vi "TRIG_conf2.vi"() -> ()   [LabVIEW 2012]
uses:
  global.vi
  <vilib>/Platform/browser.llb/Open URL in Default Browser (string).vi
panel:
  in  "additional_time":dbl=5e-06
  out "trig inhibit":dbl=100.0 min=0.0 max=999.999999999995 format="%.2p"
  out "exp cycle":dbl=100.0 min=0.0 max=999.999999999995 format="%.2f"
  out "delay cycle":dbl=100.0 min=0.0 max=999.999999999995 format="%.2f"
  in  "Close":bool
  in  "Reset TRIG":bool
  in  "write config":bool
  in  "BG cycle":dbl=100.0 format="%.2f"
  in  "mol. delay":dbl=100.0 min=0.0 max=999.999999999995 format="%.2f"
  out "Burst enable":bool=TRUE caption="Burst"
  out "Digital Waveform Graph":digitalwaveform(graph)={"t0"=timestamp(0 s since 1904-01-01), "dt"=3e-08, "Y"={"transitions"=[], "data"=array4950x4[19800 elements]}}
  in  "burst period":dbl=49.99999999999998 min=1e-07 format="%.2f"
  in  "bursts":i32=3 min=1
  in  "duration":dbl[](array[numeric])=[5.65, 5.0, 40.0, 5.0] min=0.0 format="%.3f"
  in  "start time":dbl[](array[numeric])=[0.0, 1.1, 6.6000000000000005, 6.3999999999999995] format="%.3f"
  in  "time unit":enum16{"s", "ms", "us", "ns"}(ring)=enum."us"
  in  "help":bool
  out "update front panel":bool
  # "Configure Delay Generator (TRIG)"
  # "power AMP"
  # "AWG"
  # "SWITCH"
  # "OSC"
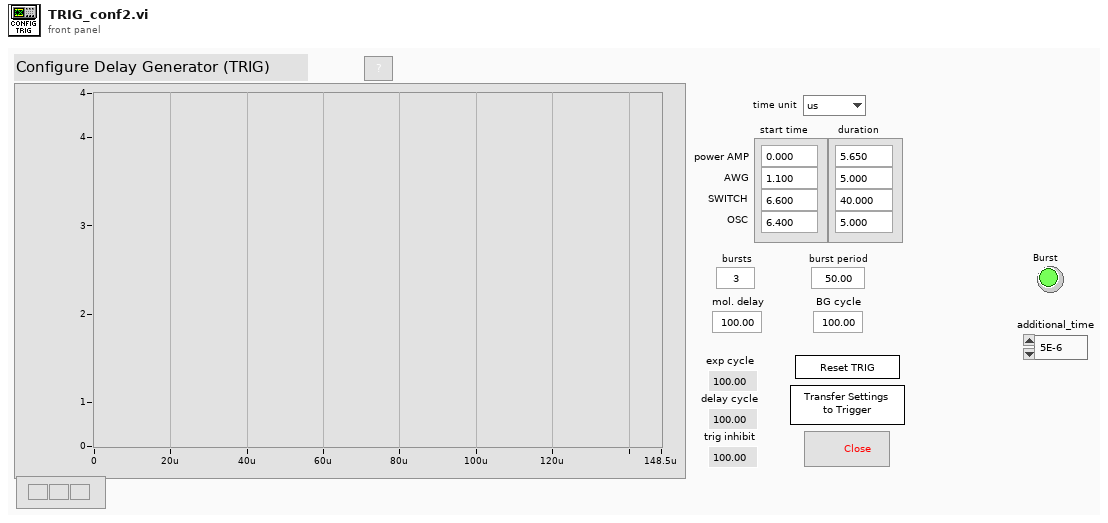
[diagram p1: front panel]
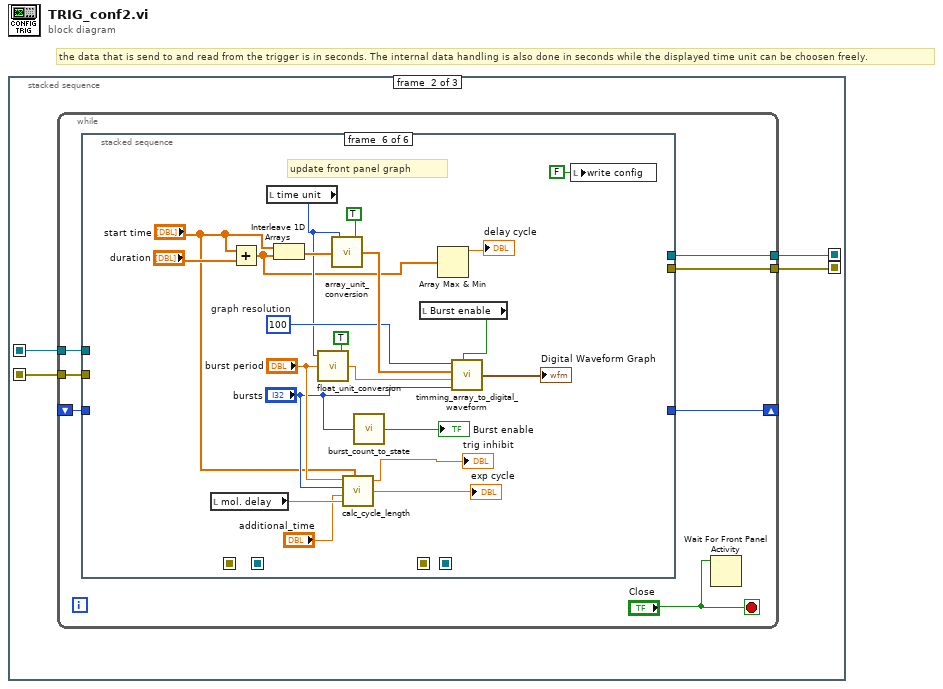
[diagram p0: block diagram]
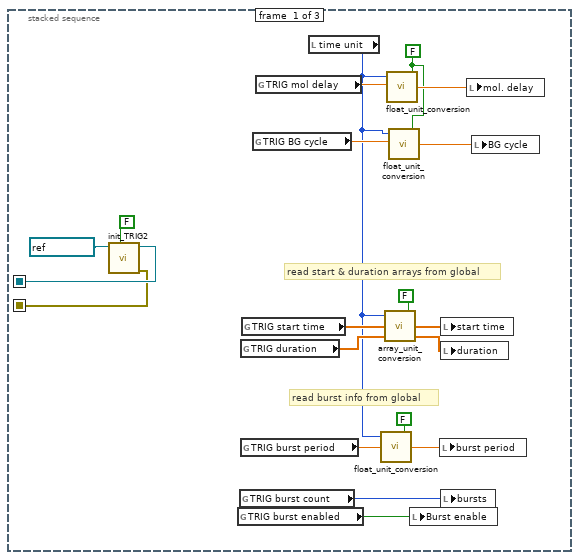
[diagram p2: hidden frame]
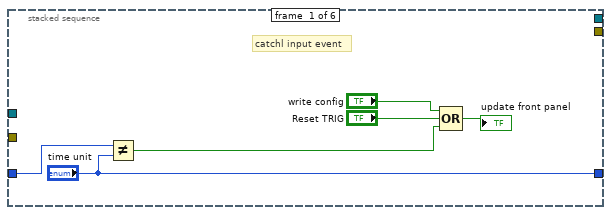
[diagram p3: hidden frame]
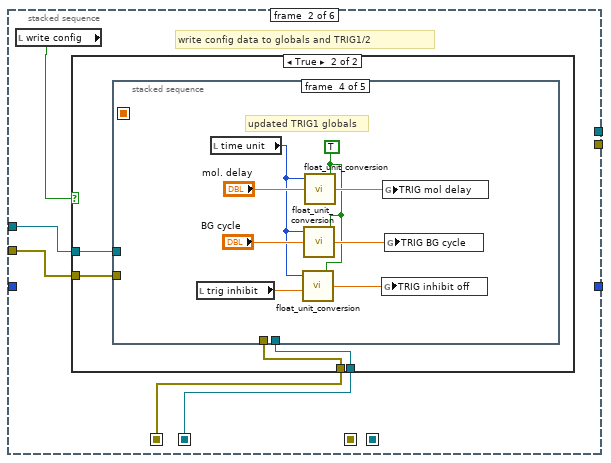
[diagram p4: hidden frame]
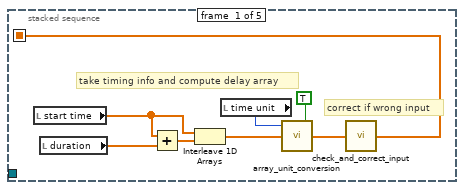
[diagram p6: hidden frame]
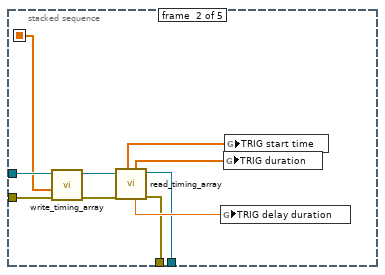
[diagram p7: hidden frame]
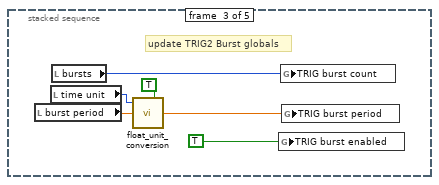
[diagram p8: hidden frame]
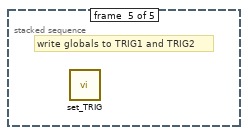
[diagram p9: hidden frame]
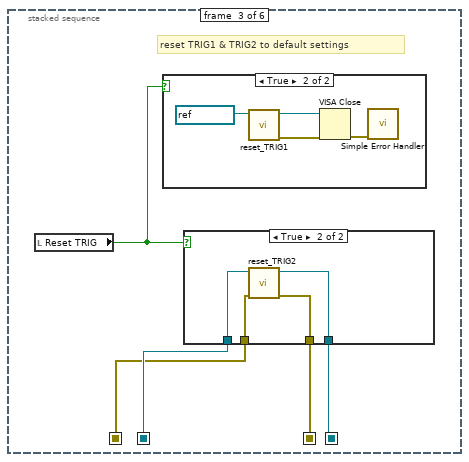
[diagram p10: hidden frame]
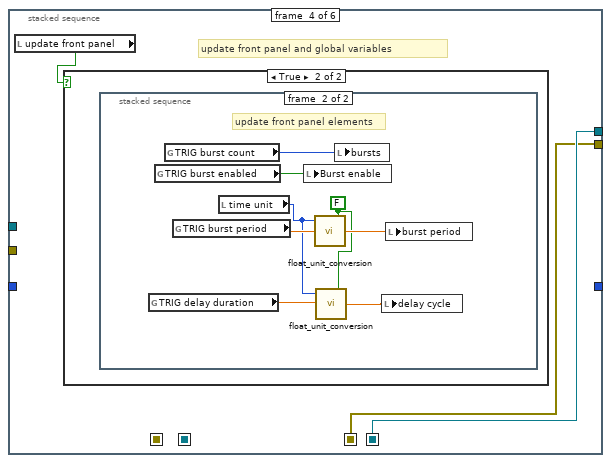
[diagram p13: hidden frame]
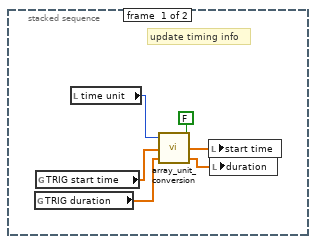
[diagram p15: hidden frame]
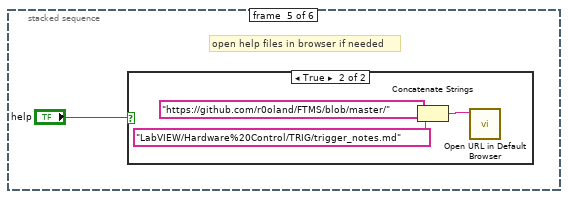
[diagram p16: hidden frame]
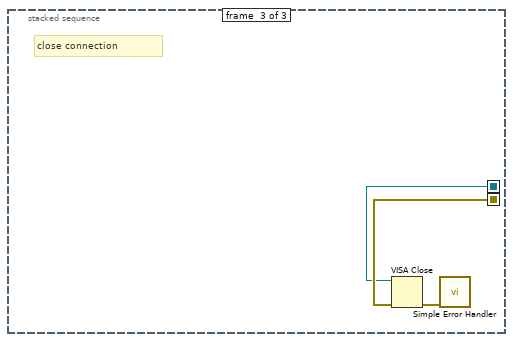
[diagram p18: hidden frame]
diagram:
  # "the data that is send to and read from the trigger is in seconds. The internal data handling is also done in seconds while the displayed time unit can be choosen freely."
  n1 = stacked-sequence {
    seq-local: [w17 _ _] -> [_ w24 _]
    seq-local: [w16 _ _] -> [_ w23 _]
    seq-local: [_ w22 _] -> [_ _ w138]
    seq-local: [_ w21 _] -> [_ _ w140]
    frame #0 {
      w2 = FALSE ("inverse")
      # "read burst info from global"
      # "read start & duration arrays from global"
      n2 = call "init_TRIG2.vi"("reset TRIG"=FALSE, "VISA resource name"=refnum<visa-resource-name> "TRIG2" ("TRIG2 resource name")) -> ("error out"=w16:errorcluster, "VISA resource name out"=w17:refnum<visa-resource-name>)  [unwired: 5 in]
      n3 = global read "global.vi" "TRIG burst enabled"() -> (w5:bool)
      n4 = global read "global.vi" "TRIG burst count"() -> (w11:i32)
      n5 = global read "global.vi" "TRIG duration"() -> (w13:dbl[])
      n6 = global read "global.vi" "TRIG burst period"() -> (w8:dbl)
      n7 = global read "global.vi" "TRIG start time"() -> (w15:dbl[])
      n8 = global read "global.vi" "TRIG BG cycle"() -> (w4:dbl)
      n9 = global read "global.vi" "TRIG mol delay"() -> (w7:dbl)
      n10 = local read "time unit"() -> (w3:enum16{"s", "ms", "us", "ns"})
      n11 = call "float_unit_conversion.vi"("inverse function (arb. unit to s)?"=FALSE, "time"=w8, "time unit"=w3) -> ("converted time"=w9:dbl)  [unwired: 2 in]
      n12 = call "array_unit_conversion.vi"("inverse function (arb. unit to s)?"=FALSE, "delay array 2"=w13, "delay array"=w15, "time unit"=w3) -> ("output 2"=w12:dbl[], "output"=w14:dbl[])
      n13 = call "float_unit_conversion.vi"("inverse function (arb. unit to s)?"=w2, "time"=w7, "time unit"=w3) -> ("converted time"=w6:dbl)  [unwired: 2 in]
      n14 = call "float_unit_conversion.vi"("inverse function (arb. unit to s)?"=w2, "time"=w4, "time unit"=w3) -> ("converted time"=w1:dbl)  [unwired: 2 in]
      n15 = local write "Burst enable"(w5) -> ()
      n16 = local write "burst period"(w9) -> ()
      n17 = local write "start time"(w14) -> ()
      n18 = local write "duration"(w12) -> ()
      n19 = local write "bursts"(w11) -> ()
      n20 = local write "mol. delay"(w6) -> ()
      n21 = local write "BG cycle"(w1) -> ()
    }
    frame #1 {
      n22 = while {
        tunnel: w23 -> [w29]
        tunnel: [w31] -> w22
        tunnel: [w30] -> w21
        tunnel: w24 -> [w28]
        shift-right: [w27] -> _
        shift-left: _ -> [w26]
        stop <- "Close" stop-if-true
        n23 = stacked-sequence {
          seq-local: [_ w38 _ _ _ _] -> [_ _ w81 _ _ _]
          seq-local: [_ w39 _ _ _ _] -> [_ _ w82 _ _ _]
          seq-local: [_ _ w84 _ _ _] -> [_ _ _ w96 _ _]
          seq-local: [_ _ w85 _ _ _] -> [_ _ _ w97 _ _]
          tunnel: w28 -> [_ w41 _ _ _ _]
          tunnel: w29 -> [_ w40 _ _ _ _]
          tunnel: [_ _ _ w96 _ _] -> w30
          tunnel: [_ _ _ w97 _ _] -> w31
          tunnel: ["time unit" _ _ _ _ _] -> w27
          tunnel: w26 -> [w34 _ _ _ _ _]
          frame #0 {
            # "catchl input event"
            n24 = Not Equal?(x=w34, y="time unit") -> (x != y?=w35:bool)
            n25 = Compound Arithmetic op=OR("write config", "Reset TRIG", w35) -> (→"update front panel":bool)
          }
          frame #1 {
            # "write config data to globals and TRIG1/2"
            n26 = local read "write config"() -> (w42:bool)
            n27 = case shown="True" w42 {
              tunnel: w41 -> [w44 w48]
              tunnel: w40 -> [w43 w47]
              tunnel: [w44 w46] -> w39
              tunnel: [w43 w45] -> w38
              frame False {
              }
              frame True {
                n28 = stacked-sequence {
                  seq-local: [w49 _ _ _ _] -> [_ w59 _ _ _]
                  tunnel: w48 -> [_ w63 _ _ _]
                  tunnel: w47 -> [_ w62 _ _ _]
                  tunnel: [_ w58 _ _ _] -> w46
                  tunnel: [_ w57 _ _ _] -> w45
                  frame #0 {
                    # "correct if wrong input"
                    # "take timing info and compute delay array"
                    n29 = local read "start time"() -> (w51:dbl[])
                    n30 = local read "duration"() -> (w50:dbl[])
                    n31 = Add(x=w51, y=w50) -> (x+y=w55:dbl[])
                    n32 = Interleave 1D Arrays(w51, w55) -> (w53:dbl[])
                    n33 = local read "time unit"() -> (w52:enum16{"s", "ms", "us", "ns"})
                    n34 = call "array_unit_conversion.vi"("inverse function (arb. unit to s)?"=TRUE, "delay array"=w53, "time unit"=w52) -> ("output"=w56:dbl[])  [unwired: 1 in, 1 out]
                    n35 = call "check_and_correct_input.vi"("delay array"=w56) -> ("corrrected delay array"=w49:dbl[])  [unwired: 4 in]
                  }
                  frame #1 {
                    n36 = call "write_timing_array.vi"("error in"=w62, "delay array"=w59, "VISA resource in"=w63) -> ("error out 2"=w60:errorcluster, "VISA resource out"=w61:refnum<visa-resource-name>)  [unwired: 3 in]
                    n37 = call "read_timing_array.vi"("error in"=w60, "VISA resource in"=w61) -> ("error out 2"=w57:errorcluster, "VISA resource out"=w58:refnum<visa-resource-name>, "delay duration"=w66:dbl, "duration"=w64:dbl[], "start time"=w65:dbl[])  [unwired: 5 in]
                    n38 = global write "global.vi" "TRIG delay duration"(w66) -> ()
                    n39 = global write "global.vi" "TRIG duration"(w64) -> ()
                    n40 = global write "global.vi" "TRIG start time"(w65) -> ()
                  }
                  frame #2 {
                    # "update TRIG2 Burst globals"
                    n41 = local read "burst period"() -> (w72:dbl)
                    n42 = local read "time unit"() -> (w70:enum16{"s", "ms", "us", "ns"})
                    n43 = local read "bursts"() -> (w68:i32)
                    n44 = call "float_unit_conversion.vi"("inverse function (arb. unit to s)?"=TRUE, "time"=w72, "time unit"=w70) -> ("converted time"=w69:dbl)  [unwired: 2 in]
                    n45 = global write "global.vi" "TRIG burst enabled"(TRUE ("TRIG burst enabled")) -> ()
                    n46 = global write "global.vi" "TRIG burst count"(w68) -> ()
                    n47 = global write "global.vi" "TRIG burst period"(w69) -> ()
                  }
                  frame #3 {
                    w75 = TRUE ("inverse")
                    # "updated TRIG1 globals"
                    n48 = local read "trig inhibit"() -> (w73:dbl)
                    n49 = local read "time unit"() -> (w76:enum16{"s", "ms", "us", "ns"})
                    n50 = call "float_unit_conversion.vi"("inverse function (arb. unit to s)?"=w75, "time"=w73, "time unit"=w76) -> ("converted time"=w74:dbl)  [unwired: 2 in]
                    n51 = call "float_unit_conversion.vi"("inverse function (arb. unit to s)?"=w75, "time"="BG cycle", "time unit"=w76) -> ("converted time"=w77:dbl)  [unwired: 2 in]
                    n52 = call "float_unit_conversion.vi"("inverse function (arb. unit to s)?"=w75, "time"="mol. delay", "time unit"=w76) -> ("converted time"=w79:dbl)  [unwired: 2 in]
                    n53 = global write "global.vi" "TRIG inhibit off"(w74) -> ()
                    n54 = global write "global.vi" "TRIG mol delay"(w79) -> ()
                    n55 = global write "global.vi" "TRIG BG cycle"(w77) -> ()
                  }
                  frame #4 {
                    # "write globals to TRIG1 and TRIG2"
                    n56 = call "set_TRIG.vi"() -> ()  [unwired: 12 in]
                  }
                }
              }
            }
          }
          frame #2 {
            # "reset TRIG1 & TRIG2 to default settings"
            n57 = local read "Reset TRIG"() -> (w83:bool)
            n58 = case shown="True" w83 {
              frame False {
              }
              frame True {
                n59 = call "reset_TRIG1.vi"("VISA resource name"=refnum<visa-resource-name> "TRIG1") -> ("error out"=w86:errorcluster, "VISA resource name out"=w87:refnum<visa-resource-name>)  [unwired: 9 in]
                n60 = VISA Close(VISA resource name=w87, error in (no error)=w86) -> (error out=w88:errorcluster)
                n61 = call <vilib>:"Simple Error Handler.vi"("error in (no error)"=w88) -> ()  [unwired: 4 in, 5 out]
              }
            }
            n62 = case shown="True" w83 {
              tunnel: w81 -> [w90 w92]
              tunnel: w82 -> [w91 w93]
              tunnel: [w91 w94] -> w85
              tunnel: [w90 w95] -> w84
              frame False {
              }
              frame True {
                n63 = call "reset_TRIG2.vi"("error in (no error)"=w92, "VISA resource name"=w93) -> ("error out"=w95:errorcluster, "VISA resource name out"=w94:refnum<visa-resource-name>)  [unwired: 8 in]
              }
            }
          }
          frame #3 {
            # "update front panel and global variables"
            n64 = local read "update front panel"() -> (w98:bool)
            n65 = case shown="True" w98 {
              frame False {
              }
              frame True {
                n66 = stacked-sequence {
                  frame #0 {
                    # "update timing info"
                    n67 = global read "global.vi" "TRIG duration"() -> (w99:dbl[])
                    n68 = global read "global.vi" "TRIG start time"() -> (w100:dbl[])
                    n69 = local read "time unit"() -> (w101:enum16{"s", "ms", "us", "ns"})
                    n70 = call "array_unit_conversion.vi"("inverse function (arb. unit to s)?"=FALSE, "delay array 2"=w99, "delay array"=w100, "time unit"=w101) -> ("output 2"=w102:dbl[], "output"=w103:dbl[])
                    n71 = local write "start time"(w103) -> ()
                    n72 = local write "duration"(w102) -> ()
                  }
                  frame #1 {
                    w108 = FALSE ("inverse function (arb. unit to s)?")
                    # "update front panel elements"
                    n73 = global read "global.vi" "TRIG delay duration"() -> (w106:dbl)
                    n74 = global read "global.vi" "TRIG burst enabled"() -> (w109:bool)
                    n75 = global read "global.vi" "TRIG burst count"() -> (w112:i32)
                    n76 = global read "global.vi" "TRIG burst period"() -> (w111:dbl)
                    n77 = local read "time unit"() -> (w107:enum16{"s", "ms", "us", "ns"})
                    n78 = local write "Burst enable"(w109) -> ()
                    n79 = call "float_unit_conversion.vi"("inverse function (arb. unit to s)?"=w108, "time"=w111, "time unit"=w107) -> ("converted time"=w110:dbl)  [unwired: 2 in]
                    n80 = call "float_unit_conversion.vi"("inverse function (arb. unit to s)?"=w108, "time"=w106, "time unit"=w107) -> ("converted time"=w105:dbl)  [unwired: 2 in]
                    n81 = local write "bursts"(w112) -> ()
                    n82 = local write "delay cycle"(w105) -> ()
                    n83 = local write "burst period"(w110) -> ()
                  }
                }
              }
            }
          }
          frame #4 {
            # "open help files in browser if needed"
            n84 = case shown="True" "help" {
              frame False {
              }
              frame True {
                n85 = Concatenate Strings("https://github.com/r0oland/FTMS/blob/master/" ("string"), "LabVIEW/Hardware%20Control/TRIG/trigger_notes.md" ("string")) -> (w116:string)
                n86 = call-poly <vilib>:"Open URL in Default Browser.vi"("URL"=w116) -> ()  [unwired: 5 in, 2 out]
              }
            }
          }
          frame #5 {
            w134 = 100  # graph resolution
            # "update front panel graph"
            n87 = local read "mol. delay"() -> (w122:dbl)
            n88 = Add(x="start time", y="duration") -> (x+y=w120:dbl[])
            n89 = local read "time unit"() -> (w130:enum16{"s", "ms", "us", "ns"})
            n90 = Interleave 1D Arrays("start time", w120) -> (w136:dbl[])
            n91 = call "float_unit_conversion.vi"("inverse function (arb. unit to s)?"=TRUE, "time"="burst period", "time unit"=w130) -> ("converted time"=w129:dbl)  [unwired: 2 in]
            n92 = call "array_unit_conversion.vi"("inverse function (arb. unit to s)?"=TRUE, "delay array"=w136, "time unit"=w130) -> ("output"=w135:dbl[])  [unwired: 1 in, 1 out]
            n93 = call "calc_cycle_length.vi"("burst period"="burst period", "start time"="start time", "burst amount"="bursts", "additional_time"="additional_time", "mol delay"=w122) -> ("trig inhibit"=→"trig inhibit":dbl, "exp cycle duration"=→"exp cycle":dbl)  [unwired: 2 in]
            n94 = call "burst_count_to_state.vi"("burst count"="bursts") -> ("Burst On"=→"Burst enable":bool)  [unwired: 4 in]
            n95 = local read "Burst enable"() -> (w127:bool)
            n96 = Array Max & Min(array=w120) -> (max value=→"delay cycle":dbl)  [unwired: 3 out]
            n97 = call "timming_array_to_digital_waveform.vi"("resolution"=w134, "delay array"=w135, "burst period"=w129, "burst count"="bursts", "Burst?"=w127) -> ("digital waveform"=→"Digital Waveform Graph":digitalwaveform)  [unwired: 2 in]
            n98 = local write "write config"(FALSE ("write config")) -> ()
          }
        }
        n99 = Wait For Front Panel Activity(3:"Close") -> ()  [unwired: 2 in, 1 out]
      }
    }
    frame #2 {
      # "close connection"
      n100 = VISA Close(VISA resource name=w138, error in (no error)=w140) -> (error out=w139:errorcluster)
      n101 = call <vilib>:"Simple Error Handler.vi"("error in (no error)"=w139) -> ()  [unwired: 4 in, 5 out]
    }
  }
